vi "ErrorsEqual.vi"(4 "Error in 2":errorcluster, 5 "Error in 1":errorcluster) -> (1 "Errors equal?":bool)   [LabVIEW 2017, in "GPError.lvlib"]
doc: "Compares two error wires.\n\n<B>Errors equal?</B> will be True only if <B>Error in 1</B> is identical with <B>Error in 2</B>.\n\nTwo errors are considered equal only if their code, status, source and description fields are all identical. Two errors that differ only in timestamp (the AppendTimestamp, SetError, and SetWarning functions can include a timestamp) are considered equal as well however.\n\nThis function supports comparison of appended errors, in which case each appended error in <B>Error in 1</B> must match the corresponding appended error in <B>Error in 2</B> for <B>Errors equal?</B> to be True.\n\nThis VI is inlined.\n\nSteen Schmidt\nGPower\n11/7 2013"
uses:
  GPError.lvlib
panel:
  # "Copyright © 2013\nSteen Schmidt, GPower\nSee enclosed license file for terms and conditions"
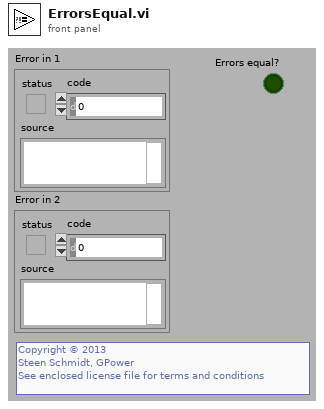
[diagram p1: front panel]
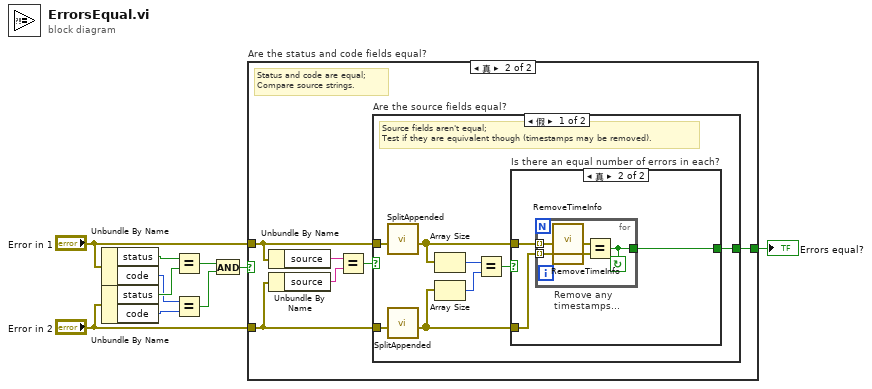
[diagram p0: block diagram]
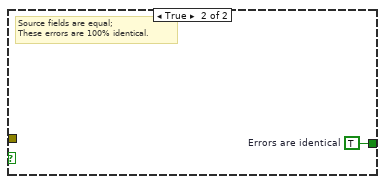
[diagram p4: hidden frame]
diagram:
  n1 = Unbundle By Name("Error in 1") -> ("status"=w7:bool, "code"=w4:i32)
  n2 = Unbundle By Name("Error in 2") -> ("status"=w6:bool, "code"=w5:i32)
  n3 = Equal?(x=w7, y=w6) -> (x = y?=w3:bool)
  n4 = Equal?(x=w4, y=w5) -> (x = y?=w2:bool)
  n5 = And(x=w3, y=w2) -> (x .and. y?=w1:bool)
  n6 = case "Are the status and code fields equal?" shown="真" w1 {
    tunnel: [_ w16] -> w10
    tunnel: "Error in 1" -> [_ w15]
    tunnel: "Error in 2" -> [_ w14]
    frame False {
      # "Status and code aren't equal;\nNo need to test further, these errors can't be equal."
    }
    frame True {
      # "Status and code are equal;\nCompare source strings."
      n7 = Unbundle By Name(w15) -> ("source"=w13:string)
      n8 = Unbundle By Name(w14) -> ("source"=w12:string)
      n9 = Equal?(x=w13, y=w12) -> (x = y?=w11:bool)
      n10 = case "Are the source fields equal?" shown="假" w11 {
        tunnel: [w19 w33] -> w16
        tunnel: w15 -> [w18 _]
        tunnel: w14 -> [w17 _]
        frame False {
          # "Source fields aren't equal;\nTest if they are equivalent though (timestamps may be removed)."
          n11 = call "SplitAppended.vi"("Appended errors in"=w18) -> ("Errors out"=w24:errorcluster[])  [unwired: 10 in]
          n12 = call "SplitAppended.vi"("Appended errors in"=w17) -> ("Errors out"=w23:errorcluster[])  [unwired: 10 in]
          n13 = Array Size(array=w24) -> (size(s)=w22:i32)
          n14 = Array Size(array=w23) -> (size(s)=w21:i32)
          n15 = Equal?(x=w22, y=w21) -> (x = y?=w20:bool)
          n16 = case "Is there an equal number of errors in each?" shown="真" w20 {
            tunnel: w24 -> [_ w27]
            tunnel: w23 -> [_ w26]
            tunnel: [_ w25] -> w19
            frame False {
              # "Different number of appended errors;\nThese errors can't be equal."
            }
            frame True {
              n17 = for "Remove any\ntimestamps..." {
                tunnel: w27 -> [w32] mode=indexing
                tunnel: w26 -> [w31] mode=indexing
                tunnel: [w28] -> w25
                stop <- w28 continue-if-true
                n18 = call "RemoveTimeInfo.vi"("Error in"=w32) -> ("Error out"=w30:errorcluster)  [unwired: 9 in, 1 out]
                n19 = call "RemoveTimeInfo.vi"("Error in"=w31) -> ("Error out"=w29:errorcluster)  [unwired: 9 in, 1 out]
                n20 = Equal?(x=w30, y=w29) -> (x = y?=w28:bool)
              }
            }
          }
        }
        frame True {
          w33 = TRUE  # Errors are identical
          # "Source fields are equal;\nThese errors are 100% identical."
        }
      }
    }
  }
  "Errors equal?" <- w10
